vi "Generic_Weighted_Stats.vi"(6 "Fluid Density":dbl=1.205, 8 "v weighting":dbl[](array[numeric]), 9 "v":dbl[](array[numeric]), 10 "u weighting":dbl[](array[numeric]), 11 "u":dbl[](array[numeric])) -> (3 "Turbulence Statistics":T1)   [LabVIEW 2011]
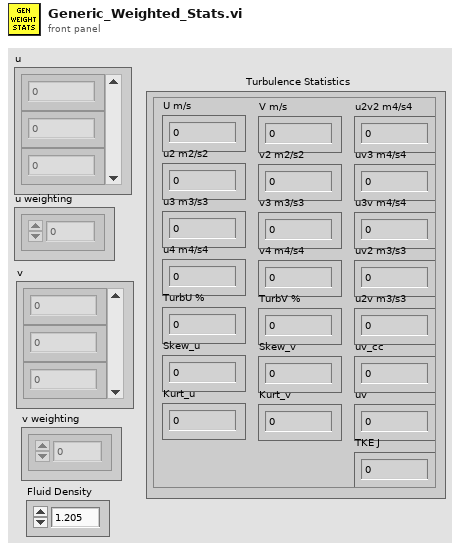
[diagram p1: front panel]
types:
  T1 = cluster{"U m/s":dbl, "u2 m2/s2":dbl, "u3 m3/s3":dbl, "u4 m4/s4":dbl, "TurbU %":dbl, "Skew_u":dbl, "Kurt_u":dbl, "V m/s":dbl, "v2 m2/s2":dbl, "v3 m3/s3":dbl, "v4 m4/s4":dbl, "TurbV %":dbl, "Skew_v":dbl, "Kurt_v":dbl, "u2v2 m4/s4":dbl, "uv3 m4/s4":dbl, "u3v m4/s4":dbl, "uv2 m3/s3":dbl, "u2v m3/s3":dbl, "uv_cc":dbl, "uv":dbl, "TKE J":dbl}
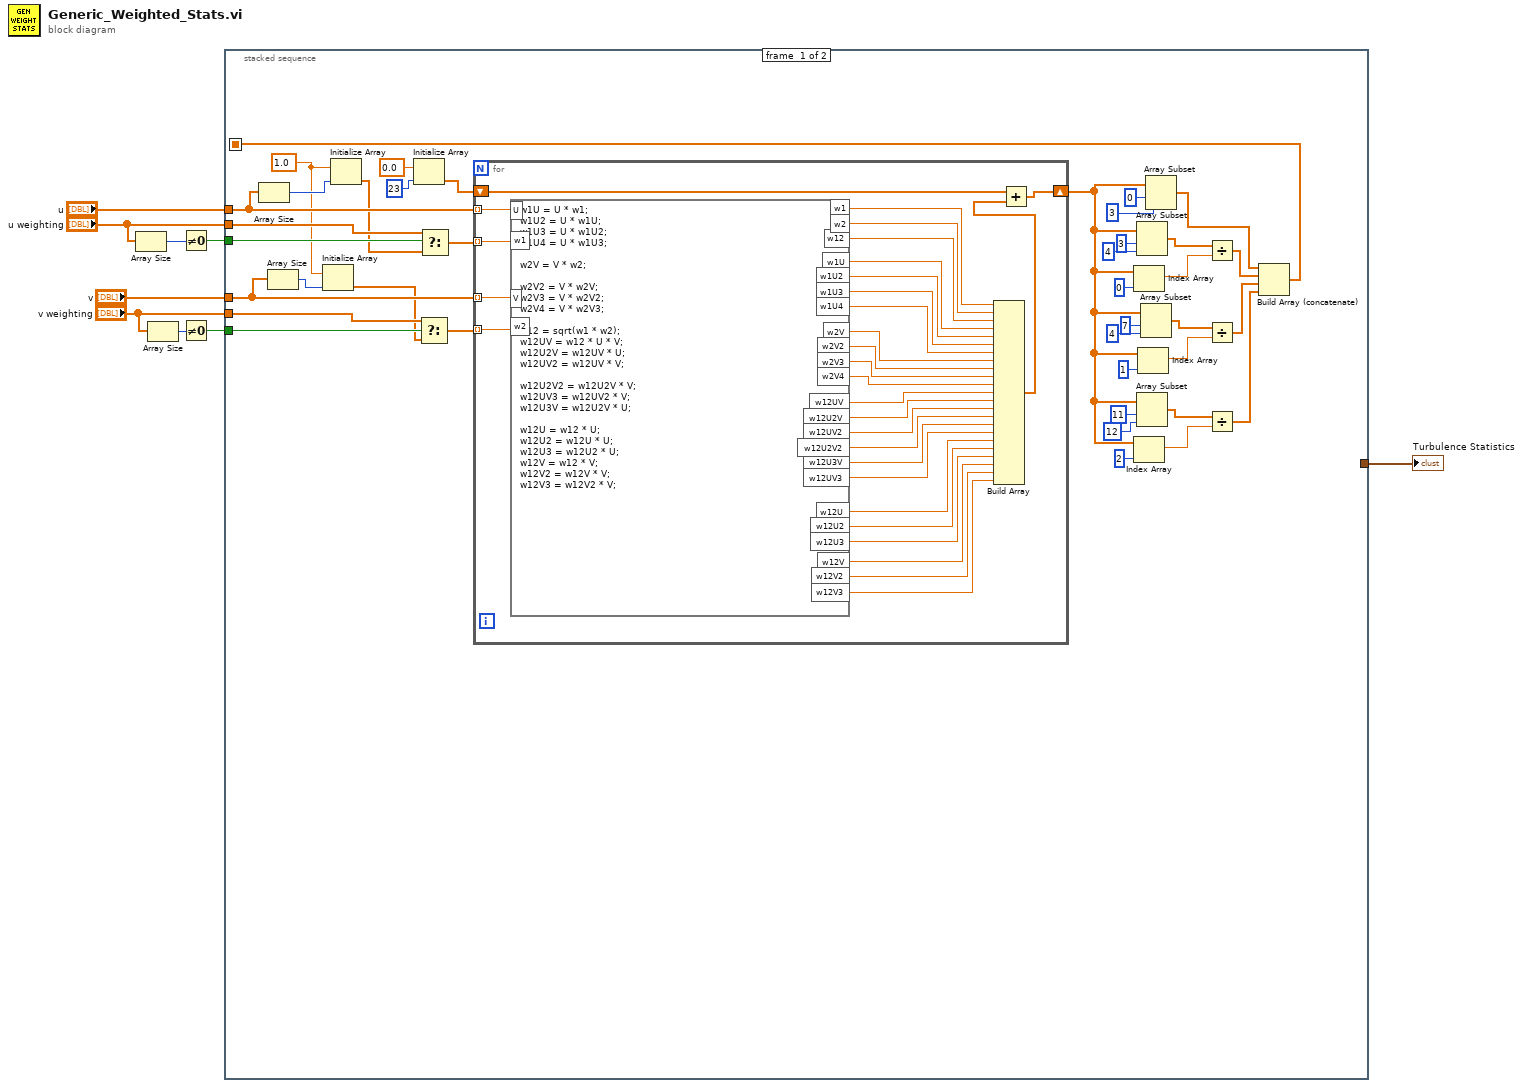
[diagram p0: block diagram]
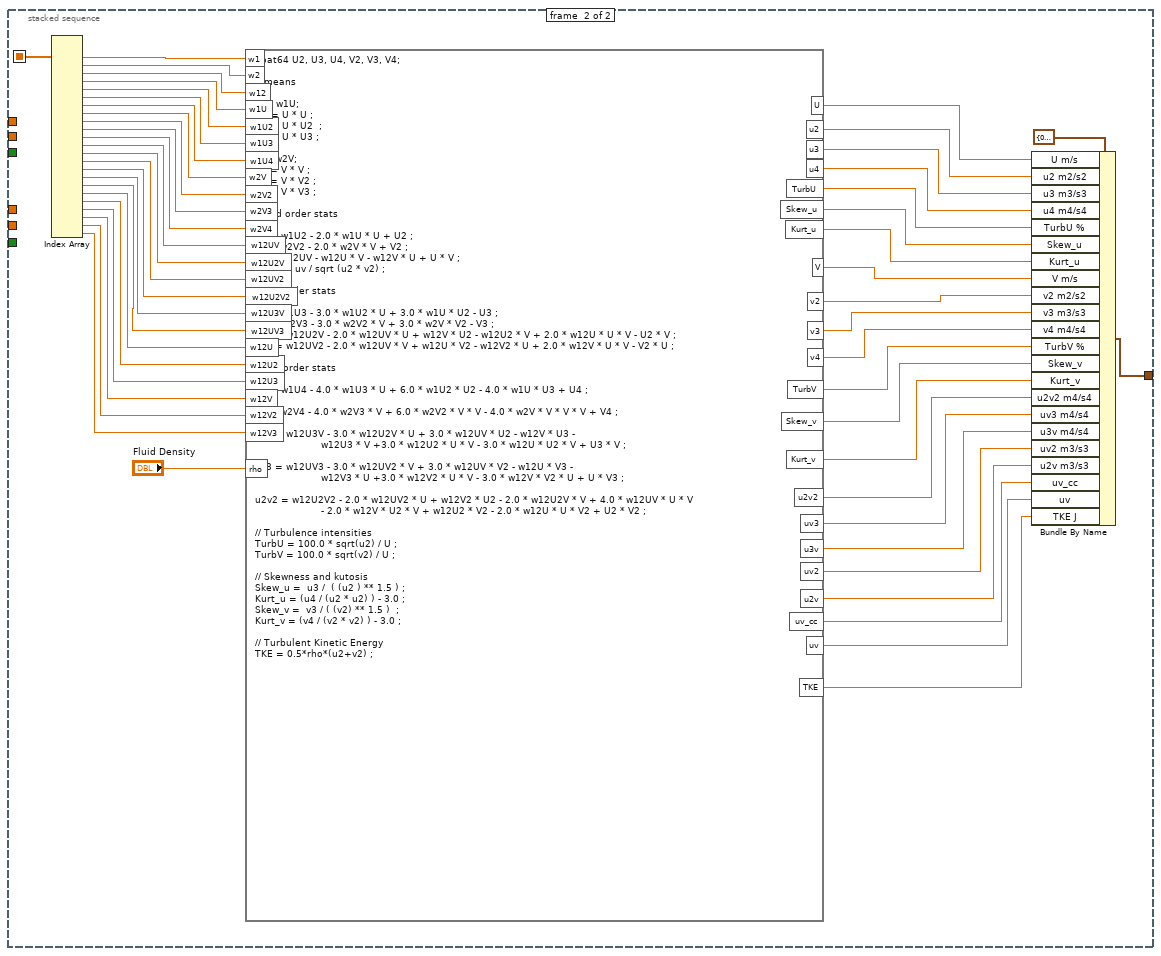
[diagram p2: hidden frame]
diagram:
  n1 = Array Size(array="u weighting") -> (size(s)=w4:i32)
  n2 = Array Size(array="v weighting") -> (size(s)=w6:i32)
  n3 = Not Equal To 0?(x=w4) -> (x != 0?=w2:bool)
  n4 = Not Equal To 0?(x=w6) -> (x != 0?=w5:bool)
  n5 = stacked-sequence {
    seq-local: [w26 _] -> [_ w101]
    tunnel: "u" -> [w16 _]
    tunnel: "v" -> [w14 _]
    tunnel: "v weighting" -> [w19 _]
    tunnel: w5 -> [w17 _]
    tunnel: "u weighting" -> [w22 _]
    tunnel: w2 -> [w21 _]
    tunnel: [_ w105] -> w1
    frame #0 {
      w12 = 1.0 ("Element Data")
      n6 = Array Size(array=w16) -> (size(s)=w15:i32)
      n7 = Array Size(array=w14) -> (size(s)=w13:i32)
      n8 = Initialize Array(w12, w13) -> (w11:dbl[])
      n9 = Initialize Array(w12, w15) -> (w10:dbl[])
      n10 = Initialize Array(0.0 ("Element Data"), 23 ("Dimension Size")) -> (w23:dbl[])
      n11 = Select(t=w19, s=w17, f=w11) -> (s? t:f=w18:dbl[])
      n12 = Select(t=w22, s=w21, f=w10) -> (s? t:f=w20:dbl[])
      n13 = for {
        shift-right: [w49] -> w27
        shift-left: w23 -> [w78]
        tunnel: w16 -> [w76] mode=indexing
        tunnel: w14 -> [w75] mode=indexing
        tunnel: w20 -> [w51] mode=indexing
        tunnel: w18 -> [w50] mode=indexing
        n14 = formula code="w1U = U * w1;\nw1U2 = U * w1U;\nw1U3 = U * w1U2;\nw1U4 = U * w1U3;\n\nw2V = V * w2;\n\nw2V2 = V * w2V;\nw2V3 = V * w2V2;\nw2V4 = V * w2V3;\n\nw12 = sqrt(w1 * w2);\nw12UV = w12 * U * V;\nw12U2V = w12UV * U;\nw12UV2 = w12UV * V;\n\nw12U2V2 = w12U2V * V;\nw12UV3 = w12UV2 * V;\nw12U3V = w12U2V * U;\n\nw12U = w12 * U;\nw12U2 = w12U * U;\nw12U3 = w12U2 * U;\nw12V = w12 * V;\nw12V2 = w12V * V;\nw12V3 = w12V2 * V;"("V"=w75, "U"=w76, "w1"=w51, "w2"=w50) -> ("w12UV"=w66:dbl, "w1U"=w74:dbl, "w2V"=w70:dbl, "w1U2"=w73:dbl, "w2V2"=w69:dbl, "w12U2V"=w65:dbl, "w12UV2"=w64:dbl, "w1U3"=w72:dbl, "w1U4"=w71:dbl, "w2V3"=w68:dbl, "w2V4"=w67:dbl, "w12U3V"=w62:dbl, "w12UV3"=w61:dbl, "w12U2V2"=w63:dbl, "w12U"=w57:dbl, "w12U2"=w56:dbl, "w12U3"=w55:dbl, "w12V"=w54:dbl, "w12V2"=w53:dbl, "w12V3"=w52:dbl, "w12"=w60:dbl, "w1"=w59:dbl, "w2"=w58:dbl)
        n15 = Build Array(w59, w58, w60, w74, w73, w72, w71, w70, w69, w68, w67, w66, w65, w64, w63, w62, w61, w57, w56, w55, w54, w53, w52) -> (w77:dbl[])
        n16 = Add(x=w78, y=w77) -> (x+y=w49:dbl[])
      }
      n17 = Index Array(array=w27, index=0 ("Index")) -> (element=w45:dbl)
      n18 = Index Array(array=w27, index=2 ("Index")) -> (element=w35:dbl)
      n19 = Array Subset(array=w27, index=3 ("Array Index"), length=4) -> (w46:dbl[])
      n20 = Array Subset(array=w27, index=11 ("Array Index"), length=12) -> (w36:dbl[])
      n21 = Index Array(array=w27, index=1 ("Index")) -> (element=w42:dbl)
      n22 = Array Subset(array=w27, index=7 ("Array Index"), length=4) -> (w41:dbl[])
      n23 = Array Subset(array=w27, index=0, length=3) -> (w28:dbl[])
      n24 = Divide(x=w46, y=w45) -> (x/y=w33:dbl[])
      n25 = Divide(x=w41, y=w42) -> (x/y=w32:dbl[])
      n26 = Divide(x=w36, y=w35) -> (x/y=w31:dbl[])
      n27 = Build Array (concatenate)(w28, w33, w32, w31) -> (w26:dbl[])
    }
    frame #1 {
      n28 = Index Array(array=w101) -> (element #1=w127:dbl, element #2=w100:dbl, element #3=w99:dbl, element #4=w98:dbl, element #5=w97:dbl, element #6=w96:dbl, element #7=w95:dbl, element #8=w94:dbl, element #9=w93:dbl, element #10=w92:dbl, element #11=w91:dbl, element #12=w90:dbl, element #13=w89:dbl, element #14=w88:dbl, element #15=w87:dbl, element #16=w86:dbl, element #17=w85:dbl, element #18=w84:dbl, element #19=w83:dbl, element #20=w82:dbl, element #21=w81:dbl, element #22=w80:dbl, element #23=w79:dbl)  [unwired: 23 in]
      n29 = formula code="float64 U2, U3, U4, V2, V3, V4;\n\n// means\n\nU = w1U;\nU2 = U * U ;\nU3 = U * U2  ;\nU4 = U * U3 ;\n\nV = w2V;\nV2 = V * V ;\nV3 = V * V2 ;\nV4 = V * V3 ;\n\n// 2nd order stats\n\nu2 = w1U2 - 2.0 * w1U * U + U2 ;\nv2 = w2V2 - 2.0 * w2V * V + V2 ;\nuv = w12UV - w12U * V - w12V * U + U * V ;\nuv_cc = uv / sqrt (u2 * v2) ;\n\n// 3rd order stats\n\nu3 = w1U3 - 3.0 * w1U2 * U + 3.0 * w1U * U2 - U3 ;\nv3 =  w2V3 - 3.0 * w2V2 * V + 3.0 * w2V * V2 - V3 ;\nu2v = w12U2V - 2.0 * w12UV * U + w12V * U2 - w12U2 * V + 2.0 * w12U * U * V - U2 * V ;\nuv2 = w12UV2 - 2.0 * w12UV * V + w12U * V2 - w12V2 * U + 2.0 * w12V * U * V - V2 * U ;\n\n// 4th order stats\n\nu4 = w1U4 - 4.0 * w1U3 * U + 6.0 * w1U2 * U2 - 4.0 * w1U * U3 + U4 ;\n\nv4 = w2V4 - 4.0 * w2V3 * V + 6.0 * w2V2 * V * V - 4.0 * w2V * V * V * V + V4 ;\n\nu3v = w12U3V - 3.0 * w12U2V * U + 3.0 * w12UV * U2 - w12V * U3 - \n                      w12U3 * V +3.0 * w12U2 * U * V - 3.0 * w12U * U2 * V + U3 * V ;\n\nuv3 = w12UV3 - 3.0 * w12UV2 * V + 3.0 * w12UV * V2 - w12U * V3 - \n                      w12V3 * U +3.0 * w12V2 * U * V - 3.0 * w12V * V2 * U + U * V3 ;\n\nu2v2 = w12U2V2 - 2.0 * w12UV2 * U + w12V2 * U2 - 2.0 * w12U2V * V + 4.0 * w12UV * U * V\n                      - 2.0 * w12V * U2 * V + w12U2 * V2 - 2.0 * w12U * U * V2 + U2 * V2 ; \n\n// Turbulence intensities\nTurbU = 100.0 * sqrt(u2) / U ;\nTurbV = 100.0 * sqrt(v2) / U ;\n\n// Skewness and kutosis\nSkew_u =  u3 /  ( (u2 ) ** 1.5 ) ;\nKurt_u = (u4 / (u2 * u2) ) - 3.0 ;\nSkew_v =  v3 / ( (v2) ** 1.5 )  ;\nKurt_v = (v4 / (v2 * v2) ) - 3.0 ;\n\n// Turbulent Kinetic Energy\nTKE = 0.5*rho*(u2+v2) ;"("w1"=w127, "w2"=w100, "w12"=w99, "w1U2"=w97, "w1U3"=w96, "w1U"=w98, "w1U4"=w95, "w2V"=w94, "w2V2"=w93, "w2V4"=w91, "w2V3"=w92, "w12UV"=w90, "w12U2V"=w89, "w12UV2"=w88, "w12U2V2"=w87, "w12U3V"=w86, "w12UV3"=w85, "w12U2"=w83, "w12U3"=w82, "w12V"=w81, "w12V2"=w80, "w12U"=w84, "w12V3"=w79, "rho"="Fluid Density") -> ("uv"=w106:dbl, "U"=w126:dbl, "V"=w119:dbl, "u2"=w125:dbl, "v2"=w118:dbl, "uv_cc"=w107:dbl, "u2v"=w108:dbl, "uv2"=w109:dbl, "u3"=w124:dbl, "u4"=w123:dbl, "v3"=w117:dbl, "v4"=w116:dbl, "TurbU"=w122:dbl, "TurbV"=w115:dbl, "Skew_v"=w114:dbl, "Skew_u"=w121:dbl, "Kurt_u"=w120:dbl, "Kurt_v"=w113:dbl, "u3v"=w110:dbl, "uv3"=w111:dbl, "u2v2"=w112:dbl, "TKE"=w103:dbl)
      n30 = Bundle By Name(cluster=T1 {"U m/s"=0.0, "u2 m2/s2"=0.0, "u3 m3/s3"=0.0, "u4 m4/s4"=0.0, "TurbU %"=0.0, "Skew_u"=0.0, "Kurt_u"=0.0, "V m/s"=0.0, "v2 m2/s2"=0.0, "v3 m3/s3"=0.0, "v4 m4/s4"=0.0, "TurbV %"=0.0, "Skew_v"=0.0, "Kurt_v"=0.0, "u2v2 m4/s4"=0.0, "uv3 m4/s4"=0.0, "u3v m4/s4"=0.0, "uv2 m3/s3"=0.0, "u2v m3/s3"=0.0, "uv_cc"=0.0, "uv"=0.0, "TKE J"=0.0} ("Turbulence Statistics"), "U m/s"=w126, "u2 m2/s2"=w125, "u3 m3/s3"=w124, "u4 m4/s4"=w123, "TurbU %"=w122, "Skew_u"=w121, "Kurt_u"=w120, "V m/s"=w119, "v2 m2/s2"=w118, "v3 m3/s3"=w117, "v4 m4/s4"=w116, "TurbV %"=w115, "Skew_v"=w114, "Kurt_v"=w113, "u2v2 m4/s4"=w112, "uv3 m4/s4"=w111, "u3v m4/s4"=w110, "uv2 m3/s3"=w109, "u2v m3/s3"=w108, "uv_cc"=w107, "uv"=w106, "TKE J"=w103) -> (w105:T1)
    }
  }
  "Turbulence Statistics" <- w1
